vi "FPGA_Main_TeamUNCC.vi"() -> ()   [LabVIEW 2018]
uses:
  <vilib>/rvi/Emulation/niFpgaGetClockAttributes.vi
  <vilib>/rvi/Emulation/niFpgaSctlEmulationGetInTimedLoop.vi
  <vilib>/rvi/Emulation/niFpgaEmulationReportErrorSimple.vi
  <vilib>/rvi/eio/common/nirviEmuTemplateMethod_errors.vi
  <vilib>/rvi/interface/RandomDataEmulation/niFpgaRandomDataHandleErrors.vi
  <vilib>/rvi/Emulation/niFpgaCriticalErrorInLSC.vi
  <vilib>/eio/EIONode/EIONode.xnode
  <vilib>/rvi/DataTransferAndStorage/Container/XNode/niFpgaContainer.xnode
  <vilib>/rvi/interface/RandomDataEmulation/nirviRandomDataFpgaReadWriteTemplate.vi
panel:
  in  "sensor\nselect":bool
  out "knife edge sensor":i16
  out "photodetector":i16
  out "cap probe":i16
  in  "amplifier":bool=TRUE
  in  "voltage to v.c.":u16
  in  "stop":bool
  in  "loop time (us)":u32
  out "Overflow to RT?":bool
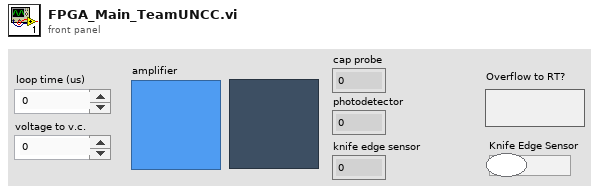
[diagram p1: front panel]
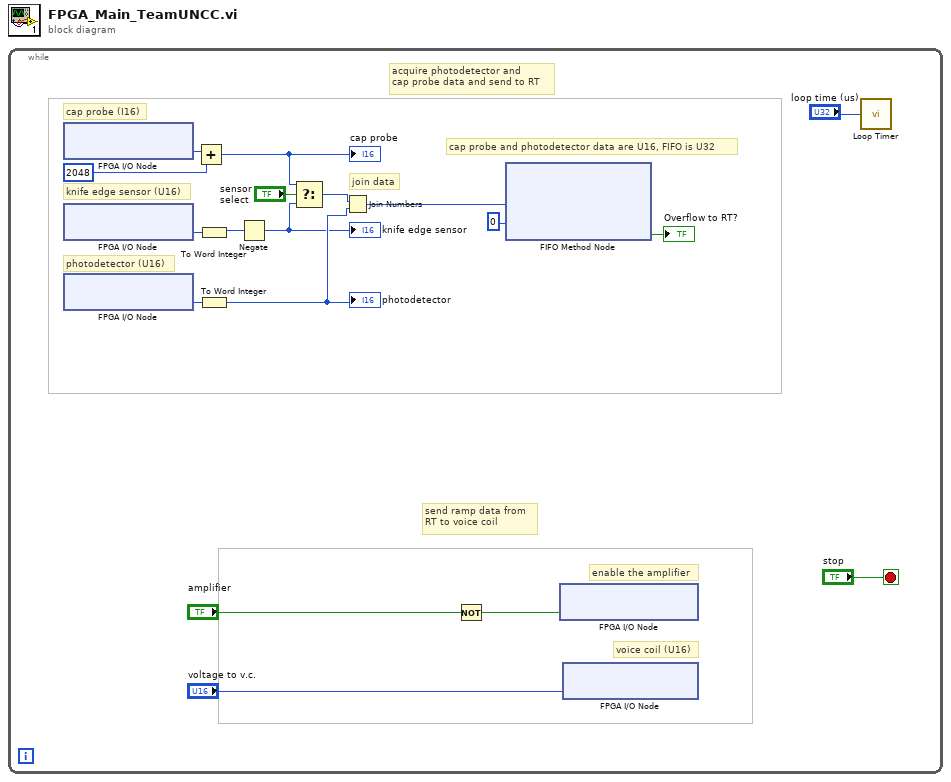
[diagram p0: block diagram]
diagram:
  n1 = while {
    stop <- "stop" stop-if-true
    # "knife edge sensor (U16)"
    # "enable the amplifier"
    # "voice coil (U16)"
    # "send ramp data from\nRT to voice coil"
    # "cap probe and photodetector data are U16, FIFO is U32"
    # "join data"
    # "photodetector (U16)"
    # "cap probe (I16)"
    # "acquire photodetector and\ncap probe data and send to RT"
    n2 = xnode "FPGA I/O Node"() -> ("ConnectorC/AI0"=w13:i16)  [unwired: 1 in, 1 out]
    n3 = xnode "FPGA I/O Node"() -> ("ConnectorA/AI1"=w8:u16)  [unwired: 1 in, 1 out]
    n4 = xnode "FPGA I/O Node"() -> ("ConnectorA/AI0"=w5:u16)  [unwired: 1 in, 1 out]
    n5 = Add(x=w13, y=i16 2048) -> (x+y=w7:i16)
    "cap probe" <- w7
    n6 = To Word Integer(number=w8) -> (16bit integer=w6:i16)
    n7 = To Word Integer(number=w5) -> (16bit integer=w2:i16)
    "photodetector" <- w2
    n8 = Negate(x=w6) -> (-x=w1:i16)
    "knife edge sensor" <- w1
    n9 = Select(t=w7, s="sensor\nselect", f=w1) -> (s? t:f=w4:i16)
    n10 = Join Numbers(hi=w4, lo=w2) -> ((hi.lo)=w3:u32)
    n11 = Not(x="amplifier") -> (.not. x?=w10:bool)
    n12 = xnode ("FIFO Method Node")("Element"=w3, "Timeout"=0) -> ("Timed Out?"=→"Overflow to RT?":bool)  [unwired: 1 in, 1 out]
    n13 = xnode "FPGA I/O Node"("ConnectorA/DIO0"=w10) -> ()  [unwired: 1 in, 1 out]
    n14 = xnode "FPGA I/O Node"("ConnectorA/AO0"="voltage to v.c.") -> ()  [unwired: 1 in, 1 out]
    n15 = call "Loop Timer"("Count(Ticks)"="loop time (us)") -> ()  [unwired: 1 out]
  }
